vi "GetWindowTextLength.vi"(8 "error in (no error)":errorcluster, 11 "hWnd (NULL)":T1) -> (0 "error out":errorcluster, 3 "dup hWnd":T1, 10 "Text Length":i32)   [LabVIEW 2011]
doc: "GetWindowTextLength\nThe GetWindowTextLength function retrieves the length, in characters, of the specified window's title bar text (if the window has a title bar). If the specified window is a control, the function retrieves the length of the text within the control. However, GetWindowTextLength cannot retrieve the length of the text of an edit control in another application.\n\nint GetWindowTextLength(\n HWND hWnd // handle to window or control with text\n);\n \nParameters\nhWnd \nHandle to the window or control. \nReturn Values\nIf the function succeeds, the return value is the length, in characters, of the text. Under certain conditions, this value may actually be greater than the length of the text. For more information, see the following Remarks section.\n\nIf the window has no text, the return value is zero. To get extended error information, callGetLastError. \n\nRemarks\nIf the target window is owned by the current process, GetWindowTextLength causes a WM_GETTEXTLENGTH message to be sent to the specified window or control. \n\nUnder certain conditions, the GetWindowTextLength function may return a value that is larger than the actual length of the text. This occurs with certain mixtures of ANSI and Unicode, and is due to the system allowing for the possible existence of DBCS characters within the text. The return value, however, will always be at least as large as the actual length of the text; you can thus always use it to guide buffer allocation. This behavior can occur when an application uses both ANSI functions and common dialogs, which use Unicode. It can also occur when an application uses the ANSI version of GetWindowTextLength with a window whose window procedure is Unicode, or the Unicode version of GetWindowTextLength with a window whose window procedure is ANSI. For more information on ANSI and Unicode functions, seeWin32 Function Prototypes. \n\nTo obtain the exact length of the text, use the WM_GETTEXT, LB_GETTEXT, or CB_GETLBTEXT messages, or the GetWindowText function."
uses:
  hWnd.ctl
  user32.dll
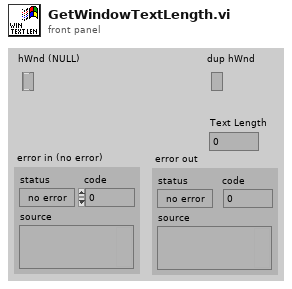
[diagram p1: front panel]
types:
  T1 = typedef "hWnd.ctl" = refnum<k1>
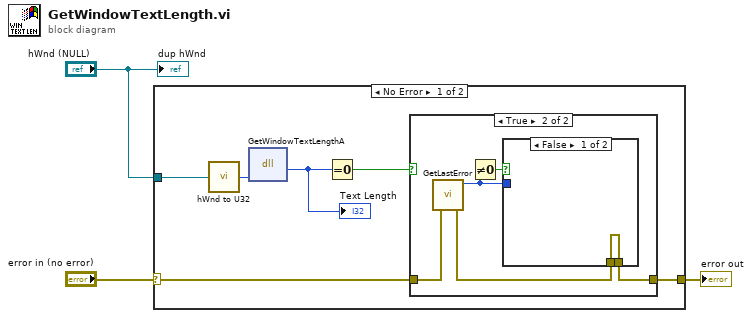
[diagram p0: block diagram]
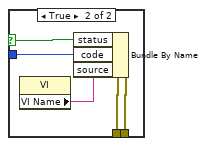
[diagram p3: hidden frame]
diagram:
  n1 = case shown="No Error" "error in (no error)" {
    selector: "error in (no error)" -> [w8 w22]
    tunnel: "hWnd (NULL)" -> [w9 _]
    tunnel: [w6 w22] -> w1
    frame No Error {
      n2 = call "hWnd to U32.vi"("hWnd"=w9) -> ("hWnd"=w5:u32)  [unwired: 4 out]
      n3 = dll-call lib="User32.dll" fn="GetWindowTextLengthA" label="GetWindowTextLength"("hWnd"=w5) -> ("TextLength"=w4:i32)  [unwired: 4 in, 2 out]
      "Text Length" <- w4
      n4 = Equal To 0?(x=w4) -> (x = 0?=w7:bool)
      n5 = case shown="True" w7 {
        tunnel: w8 -> [w10 w14]
        tunnel: [w10 w15] -> w6
        frame False {
        }
        frame True {
          n6 = call "GetLastError.vi"("error in (no error)"=w14) -> ("error out"=w13:errorcluster, "CODE"=w12:i32)  [unwired: 5 out]
          n7 = Not Equal To 0?(x=w12) -> (x != 0?=w11:bool)
          n8 = case shown="False" w11 {
            selector: w11 -> [_ w17]
            tunnel: [w16 w21] -> w15
            tunnel: w13 -> [w16 w20]
            tunnel: w12 -> [_ w18]
            frame False {
            }
            frame True {
              n9 = property class="VI"() -> ("VI Name"=w19:string)  [unwired: 2 in, 2 out]
              n10 = Bundle By Name(cluster=w20, "status"=w17, "code"=w18, "source"=w19) -> (w21:errorcluster)
            }
          }
        }
      }
    }
    frame Error {
    }
  }
  "error out" <- w1
  "dup hWnd" <- "hWnd (NULL)"
